vi "Init Command.vi"(5 "Sequencer":refnum<class "MessageQ.lvclass">, 6 "Variables":refnum<class "Variables.lvclass">, 7 "VolatusAPI":refnum<class "VolatusAPI.lvclass">, 8 "error in (no error)":refnum<class "MultiErrors.lvclass">, 10 "Command Config":refnum<class "Command Config.lvclass">, 11 "Digital Command in":refnum<class "Digital Command.lvclass">) -> (0 "error out":refnum<class "MultiErrors.lvclass">, 3 "Digital Command out":T1)   [LabVIEW 2020, in "VolatusSeq.lvlib" / "Digital Command.lvclass"]
uses:
  Digital Command.lvclass
  VolatusErrorUtilities/MultiErrors/MultiErrors.lvclass
  Command.ctl
  Volatus/MessageQ/MessageQ.lvclass
  VolatusSeqConfig/Command Type.ctl
  messages/CmdDigital/Data.ctl
  messages/CmdAnalog/Data.ctl
  Send Type.ctl
  Volatus/VolatusAPI/VolatusAPI.lvclass
  VolatusSeqConfig/Command Config/Command Config.lvclass
  VolatusSeqConfig/Digital Command Config/Digital Command Config.lvclass
  Digital Command.lvclass/Digital Command.ctl
  VolatusSeqConfig/VolatusSeqConfig.lvlib
  VolatusSeq.lvlib
  messages/CmdAnalog/CmdAnalog.lvlib
  messages/CmdDigital/CmdDigital.lvlib
  Command/Command.lvclass
  Variables/Variables.lvclass
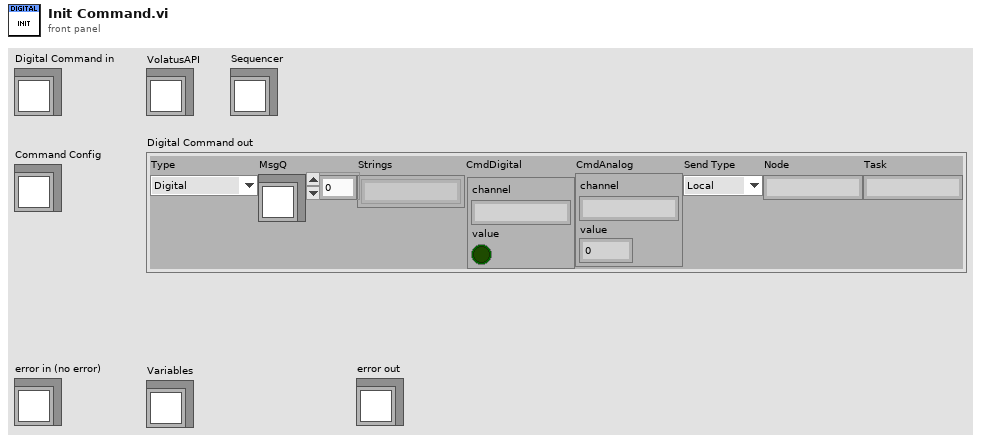
[diagram p1: front panel]
types:
  T1 = typedef "VolatusSeq.lvlib/Command.ctl" = cluster{"Type":T2, "MsgQ":refnum<class "MessageQ.lvclass">, "Strings":string[], "CmdDigital":T3, "CmdAnalog":T4, "Send Type":T5, "Node":string, "Task":string}
  T2 = typedef "VolatusSeqConfig.lvlib/Command Type.ctl" = enum16{"Digital", "Numeric", "Transition", "Stop", "StartLog", "StopLog", "Start", "Event", "Error", "HTTP"}
  T3 = typedef "CmdDigital.lvlib/Data.ctl" = cluster{"channel":string, "value":bool}
  T4 = typedef "CmdAnalog.lvlib/Data.ctl" = cluster{"channel":string, "value":dbl}
  T5 = typedef "VolatusSeq.lvlib/Send Type.ctl" = enum16{"Local", "Remote"}
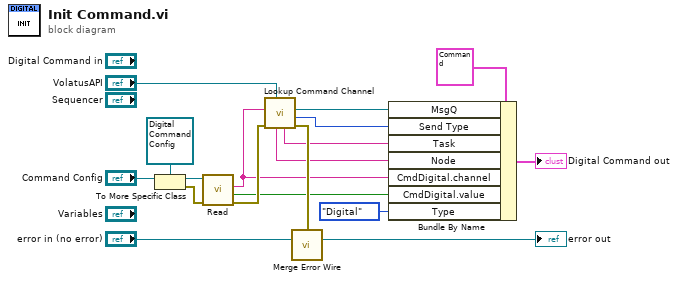
[diagram p0: block diagram]
diagram:
  n1 = To More Specific Class(target class=refnum<class "Digital Command Config.lvclass"> refnum ("VolatusSeqConfig.lvlib:Digital Command Config.lvclass"), reference="Command Config") -> (specific class reference=w14:refnum<class "Digital Command Config.lvclass">, error out=w13:errorcluster)  [unwired: 1 in]
  n2 = call "Read.vi"("error in (no error)"=w13, "Digital Command Config in"=w14) -> ("error out"=w18:errorcluster, "Command"=w8:bool, "Channel"=w6:string)  [unwired: 6 in, 1 out]
  n3 = call "Lookup Command Channel.vi"("VolatusAPI in"="VolatusAPI", "error in (no error)"=w18, "Channel Name"=w6) -> ("error out"=w17:errorcluster, "Send Type"=w3:T5, "MsgQ"=w2:refnum<class "MessageQ.lvclass">, "Owning Task"=w4:string, "Owning Node"=w5:string)  [unwired: 4 in]
  n4 = call "Merge Error Wire.vi"("error in (no error)"=w17, "MultiErrors in"="error in (no error)") -> ("MultiErrors out"=→"error out":refnum<class "MultiErrors.lvclass">)  [unwired: 13 in]
  n5 = Bundle By Name(cluster=T1 {"Type"=enum."Digital", "MsgQ"=refnum, "Strings"=[], "CmdDigital"={"channel"="", "value"=FALSE}, "CmdAnalog"={"channel"="", "value"=0.0}, "Send Type"=enum."Local", "Node"="", "Task"=""} ("Digital Command out"), "MsgQ"=w2, "Send Type"=w3, "Task"=w4, "Node"=w5, "CmdDigital.channel"=w6, "CmdDigital.value"=w8, "Type"=Command_Type."Digital") -> (→"Digital Command out":T1)
